vi "B_GetProperty.vi"(0 "reference in":refnum<class "Vision.lvclass">, 5 "error in (no error)":errorcluster) -> (14 "reference out":refnum<class "Vision.lvclass">, 15 "property":dbl, 19 "error out":errorcluster)   [LabVIEW 2023, in "Vision.lvclass"]
uses:
  Vision.lvclass
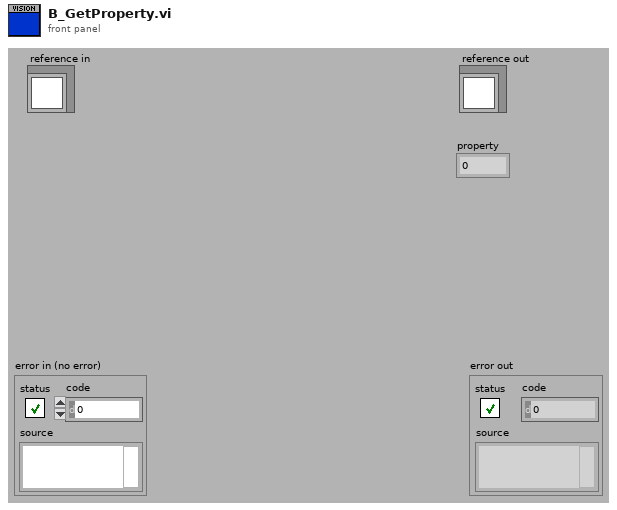
[diagram p1: front panel]
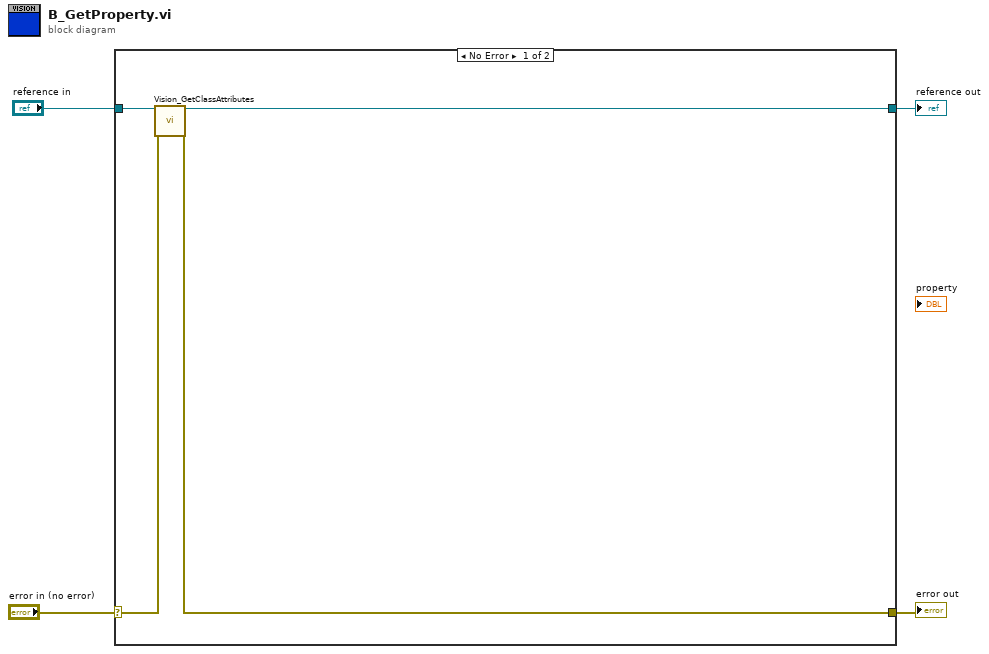
[diagram p0: block diagram]
diagram:
  n1 = case shown="No Error" "error in (no error)" {
    selector: "error in (no error)" -> [w8 w10]
    tunnel: [w7 w10] -> w3
    tunnel: [w5 w9] -> w1
    tunnel: "reference in" -> [w6 w9]
    frame No Error {
      n2 = call "Vision_GetClassAttributes.vi"("reference in"=w6, "error in (no error)"=w8) -> ("reference out"=w5:refnum<class "Vision.lvclass">, "error out"=w7:errorcluster)  [unwired: 14 in, 2 out]
    }
    frame Error {
    }
  }
  "error out" <- w3
  "reference out" <- w1
